vi "Compare Yellow With 007.vi"(8 "Error In":errorcluster, 10 "Yellow Player":dbl, 11 "007 Data":T1) -> (0 "Error Out":errorcluster, 2 "007s Turn":bool, 3 "007 Data Out":T1)   [LabVIEW 2015]
doc: "Returns true if 007 and yellow player are equal. If they are equal it means it is our turn to act."
uses:
  007 Data.ctl
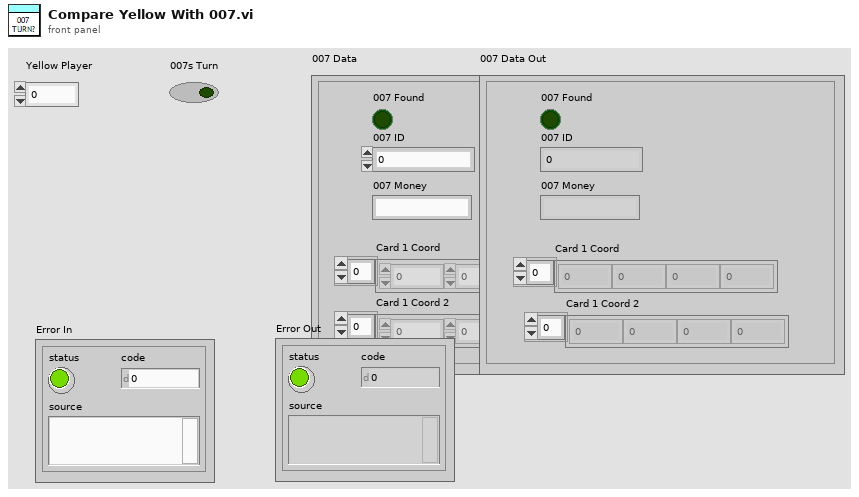
[diagram p1: front panel]
types:
  T1 = typedef "007 Data.ctl" = cluster{"007 ID":dbl, "007 Found":bool, "007 Money":string, "Card 1 Coord":i32[], "Card 1 Coord 2":i32[]}
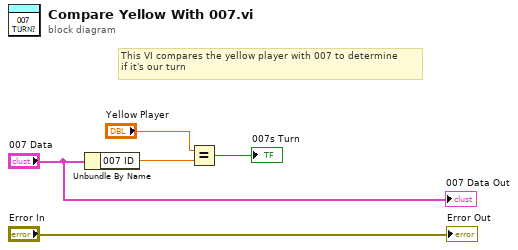
[diagram p0: block diagram]
diagram:
  # "This VI compares the yellow player with 007 to determine\nif it's our turn"
  n1 = Unbundle By Name("007 Data") -> ("007 ID"=w3:dbl)
  n2 = Equal?(x="Yellow Player", y=w3) -> (x = y?=→"007s Turn":bool)
  "Error Out" <- "Error In"
  "007 Data Out" <- "007 Data"
